vi "PC_Lens_Calibration (DONE).vi"(8 "Error In":errorcluster, 10 "Calibration File Name":string="..\\calibration.png", 11 "Grid Image Name":string="..\\grid_cal.png") -> (0 "Error Out":errorcluster)   [LabVIEW 2017]
uses:
  <vilib>/vision/Calibration.llb/Distortion Model.ctl
  <vilib>/vision/Calibration.llb/Distortion Model Types.ctl
  <vilib>/vision/NI_Vision_Development_Module.lvlib
panel:
  in  "Grid Descriptor":cluster{"X Step":sgl, "Y Step":sgl, "Unit":T1}={"X Step"=10.0, "Y Step"=10.0, "Unit"=enum."Millimeter"}
  in  "Window Size (32x32)":cluster{"SizeX":i32, "SizeY":i32}={"SizeX"=32, "SizeY"=32}
  out "Grid":T2(plugin-control)
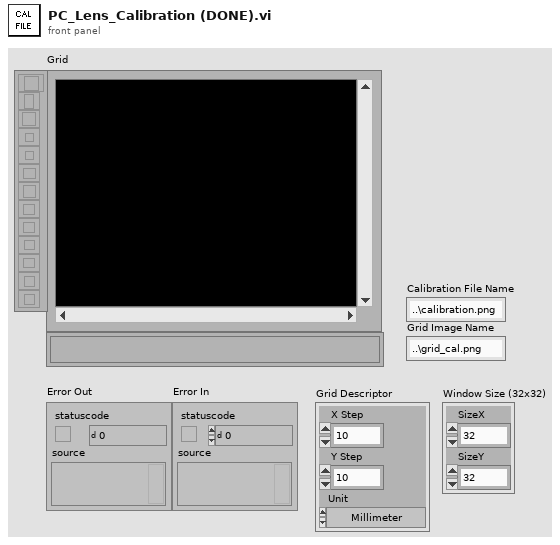
[diagram p1: front panel]
types:
  T1 = typedef "Image Unit" = enum32{"Undefined", "Angström", "Micrometer", "Millimeter", "Centimeter", "Meter", "Kilometer", "Microinch", "Inch", "Feet", "Nautical miles", "Standard miles", "Steps"}
  T2 = typedef "IMAQ Image.ctl" = refnum<image>
  T3 = typedef "Distortion Model.ctl" = cluster{"Distortion Model":T4, "Polynomial Model Setup":cluster{"Radial Coefficient":u32, "Tangential Coefficients ":bool}}
  T4 = typedef "Distortion Model Types.ctl" = i32
  T5 = typedef "Particle Parameters" = i32
  T6 = cluster{"Measurement Parameter":T5, "Range Lower Value":dbl, "Range Upper Value":dbl, "Range":bool, "Particle Parameters":bool}[]
  T7 = typedef "Calibration Reference Points.ctl" = cluster{"Pixel Coordinates":cluster{"X":dbl, "Y":dbl}[], "Real World Coordinates":cluster{"X":dbl, "Y":dbl}[], "Unit":T1, "Image Size":cluster{"X":u32, "Y":u32}}
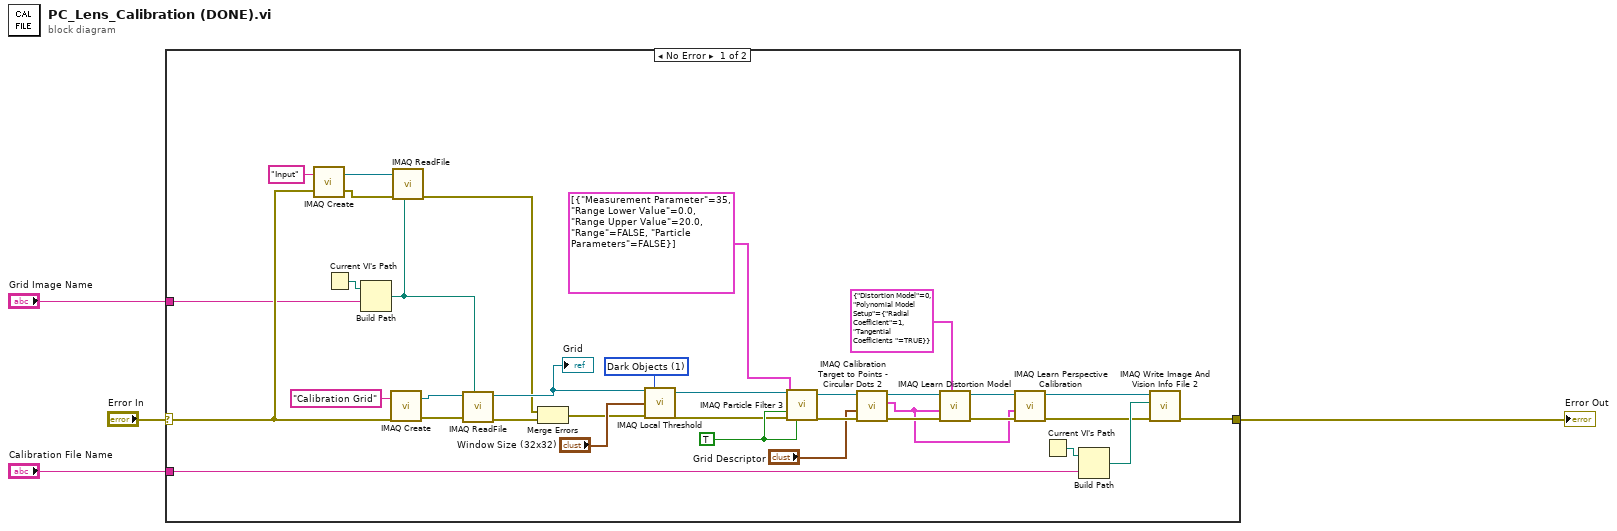
[diagram p0: block diagram]
diagram:
  n1 = case shown="No Error" "Error In" {
    selector: "Error In" -> [w13 w40]
    tunnel: [w7 w40] -> w4
    tunnel: "Calibration File Name" -> [w6 _]
    tunnel: "Grid Image Name" -> [w5 _]
    frame No Error {
      w37 = TRUE ("Keep/Remove Particles (F)")
      w38 = u32 1 items=["Bright Objects", "Dark Objects"] ("Look For (Bright Objects)")
      n2 = call "IMAQ Create"("Image Name"="Input", "error in (no error)"=w13) -> ("New Image"=w21:T2, "error out"=w24:errorcluster)  [unwired: 3 in]
      n3 = Current VI's Path() -> (path=w14:path)
      n4 = Build Path(base path=w14, name or relative path=w5) -> (appended path=w12:path)
      n5 = call "IMAQ Create"("Image Name"="Calibration Grid", "error in (no error)"=w13) -> ("New Image"=w22:T2, "error out"=w23:errorcluster)  [unwired: 3 in]
      n6 = call "IMAQ ReadFile"("File Path"=w12, "error in (no error)"=w24, "Image"=w21) -> ("error out"=w17:errorcluster)  [unwired: 4 in, 4 out]
      n7 = call "IMAQ ReadFile"("File Path"=w12, "error in (no error)"=w23, "Image"=w22) -> ("error out"=w16:errorcluster, "Image Out"=w18:T2)  [unwired: 4 in, 3 out]
      "Grid" <- w18
      n8 = Merge Errors(w17, w16) -> (w15:errorcluster)
      n9 = call "IMAQ Local Threshold"("Image Src"=w18, "Look For (Bright Objects)"=w38, "Window Size (32x32)"="Window Size (32x32)", "error in (no error)"=w15) -> ("Image Dst Out"=w35:T2, "error out"=w36:errorcluster)  [unwired: 10 in]
      n10 = call "IMAQ Particle Filter 3"("Image Src"=w35, "Selection Values"=T6 [{"Measurement Parameter"=35, "Range Lower Value"=0.0, "Range Upper Value"=20.0, "Range"=FALSE, "Particle Parameters"=FALSE}], "Keep/Remove Particles (F)"=w37, "error in (no error)"=w36, "Reject Border? (F)"=w37) -> ("Image Dst Out"=w29:T2, "error out"=w31:errorcluster)  [unwired: 8 in, 1 out]
      n11 = call "IMAQ Calibration Target to Points - Circular Dots 2"("error in (no error)"=w31, "Grid Descriptor"="Grid Descriptor", "Target Image"=w29) -> ("error out"=w32:errorcluster, "Reference Points"=w26:T7, "Target Image (dup)"=w28:T2)  [unwired: 6 in]
      n12 = call "IMAQ Learn Distortion Model"("Distortion Model Setup"=T3 {"Distortion Model"=0, "Polynomial Model Setup"={"Radial Coefficient"=1, "Tangential Coefficients "=TRUE}}, "error in (no error)"=w32, "Reference Points"=w26, "Calibration Template Image"=w28) -> ("error out"=w33:errorcluster, "Calibration Template Image Out"=w27:T2)  [unwired: 6 in]
      n13 = call "IMAQ Learn Perspective Calibration"("error in (no error)"=w33, "Reference Points"=w26, "Calibration Template Image"=w27) -> ("error out"=w8:errorcluster, "Calibration Template Image Out"=w11:T2)  [unwired: 7 in]
      n14 = Current VI's Path() -> (path=w10:path)
      n15 = Build Path(base path=w10, name or relative path=w6) -> (appended path=w9:path)
      n16 = call "IMAQ Write Image And Vision Info File 2"("error in (no error)"=w8, "File Path"=w9, "Image"=w11) -> ("error out"=w7:errorcluster)  [unwired: 7 in, 1 out]
    }
    frame Error {
    }
  }
  "Error Out" <- w4
